vi "Test_WriteValue_CheckFile_ValuePresent.vi"(8 "error in (no error)":errorcluster, 11 "TestCase in":refnum<class "TestConfigurationFileBinding.lvclass">) -> (0 "error out":errorcluster, 3 "TestCase out":refnum<class "TestConfigurationFileBinding.lvclass">)   [LabVIEW 2017, in "TestConfigurationFileBinding.lvclass"]
uses:
  TestConfigurationFileBinding.lvclass
  TestConfigurationFileBinding.lvclass/TestConfigurationFileBinding.ctl
  Source/Concrete/ConfigurationFileBinding/ConfigurationFileBinding.lvclass/ConfigurationFileBinding.ctl
  Source/Concrete/ConfigurationFileBinding/ConfigurationFileBinding.lvclass
  C:/Git/composed-transport/Source/ITransport/ITransport.lvclass
  <vilib>/Utility/error.llb/Error Cluster From Error Code.vi
  <vilib>/Utility/config.llb/Not A Config Data Refnum.vi
  <vilib>/Utility/config.llb/Read Key (I32).vi
  Source/ITransport/ITransport.lvclass
  <vilib>/Utility/config.llb/NI_LVConfig.lvlib
panel:
  out "Test File Path":path
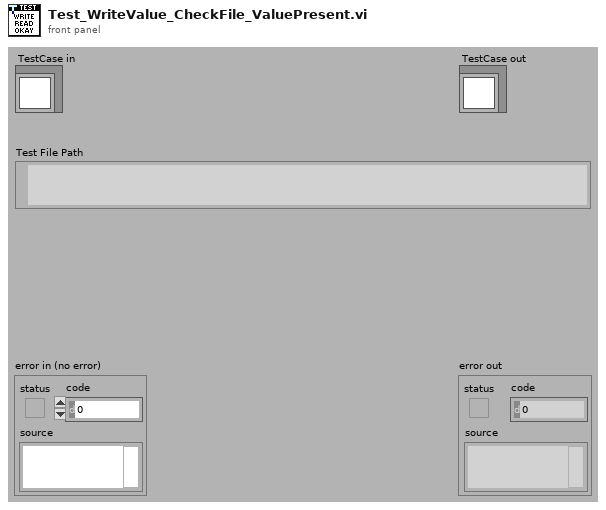
[diagram p1: front panel]
types:
  T1 = typedef "NI_LVConfig.lvlib/Config Data RefNum.ctl" = refnum<k1>
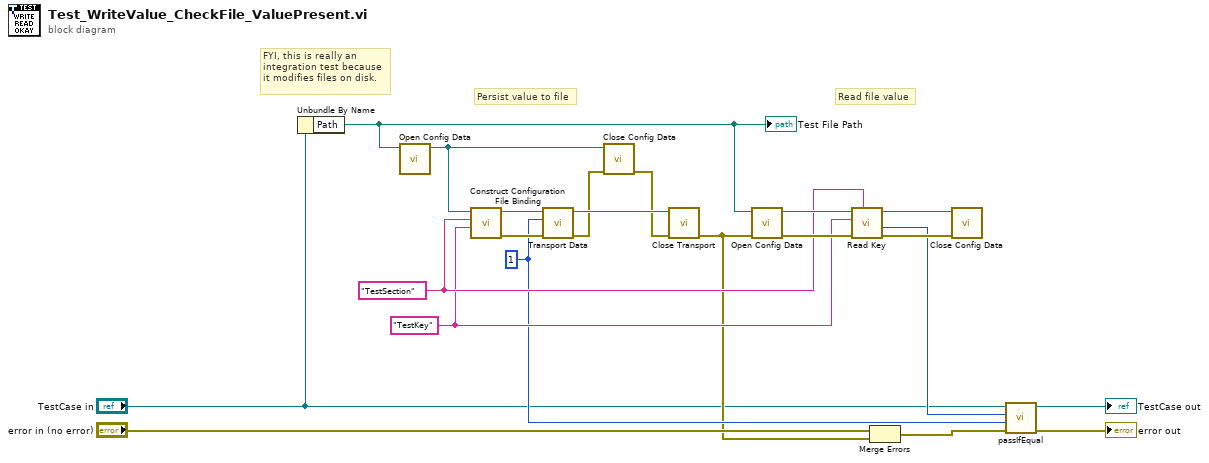
[diagram p0: block diagram]
diagram:
  w8 = "TestKey" ("Key Name")
  w9 = "TestSection" ("Section Name")
  w4 = 1 ("Test Value")
  # "FYI, this is really an\nintegration test because\nit modifies files on disk."
  # "Persist value to file"
  # "Read file value"
  n1 = Unbundle By Name("TestCase in") -> ("Path"=w1:path)
  "Test File Path" <- w1
  n2 = call <vilib>:"Open Config Data.vi"("configuration file path"=w1) -> ("refnum"=w10:T1)  [unwired: 8 in, 2 out]
  n3 = call "Construct Configuration File Binding.vi"("Key Name"=w8, "Section Name"=w9, "Config File Refnum"=w10) -> ("error out"=w20:errorcluster, "ConfigurationFileBinding"=w7:refnum<class "ConfigurationFileBinding.lvclass">)  [unwired: 7 in]
  n4 = call "Transport Data.vi"("error in (no error)"=w20, "Value"=w4, "ITransport in"=w7) -> ("error out"=w6:errorcluster, "ITransport out"=w21:refnum<class "ConfigurationFileBinding.lvclass">)  [unwired: 7 in]
  n5 = call <vilib>:"Close Config Data.vi"("error in (no error)"=w6, "refnum"=w10) -> ("error out"=w13:errorcluster)  [unwired: 8 in, 1 out]
  n6 = call-dynamic "Close Transport.vi"("error in (no error)"=w13, "ITransport in"=w21) -> ("error out"=w3:errorcluster)  [unwired: 9 in]
  n7 = call <vilib>:"Open Config Data.vi"("error in (no error)"=w3, "configuration file path"=w1) -> ("error out"=w15:errorcluster, "refnum"=w14:T1)  [unwired: 7 in, 1 out]
  n8 = call-poly <vilib>:"Read Key.vi"("section"=w9, "error in (no error)"=w15, "key"=w8, "refnum"=w14) -> ("error out"=w11:errorcluster, "value"=w5:i32, "refnum out"=w12:T1)  [unwired: 4 in, 1 out]
  n9 = Merge Errors("error in (no error)", w3) -> (w16:errorcluster)
  n10 = call <vilib>:"Close Config Data.vi"("error in (no error)"=w11, "refnum"=w12) -> ()  [unwired: 8 in, 2 out]
  n11 = call-dynamic "passIfEqual.vi"("error in (no error)"=w16, "y"=w4, "x"=w5, "TestCase in"="TestCase in") -> ("error out"=→"error out":errorcluster, "TestCase out"=→"TestCase out":refnum<class "TestConfigurationFileBinding.lvclass">)  [unwired: 6 in]
